vi "csmdoc_list_all_csm_documented_VIs.vi"() -> (3 "Array":path[](array[path]))   [LabVIEW 2017, in "csmdoc.lvlib"]
uses:
  csmdoc.lvlib
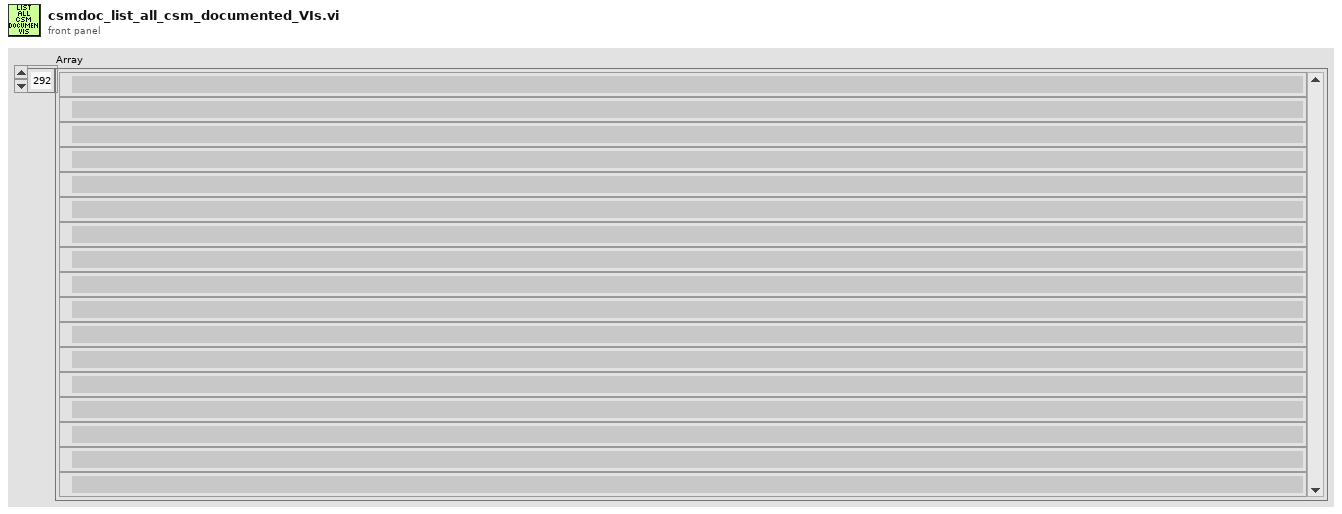
[diagram p1: front panel]
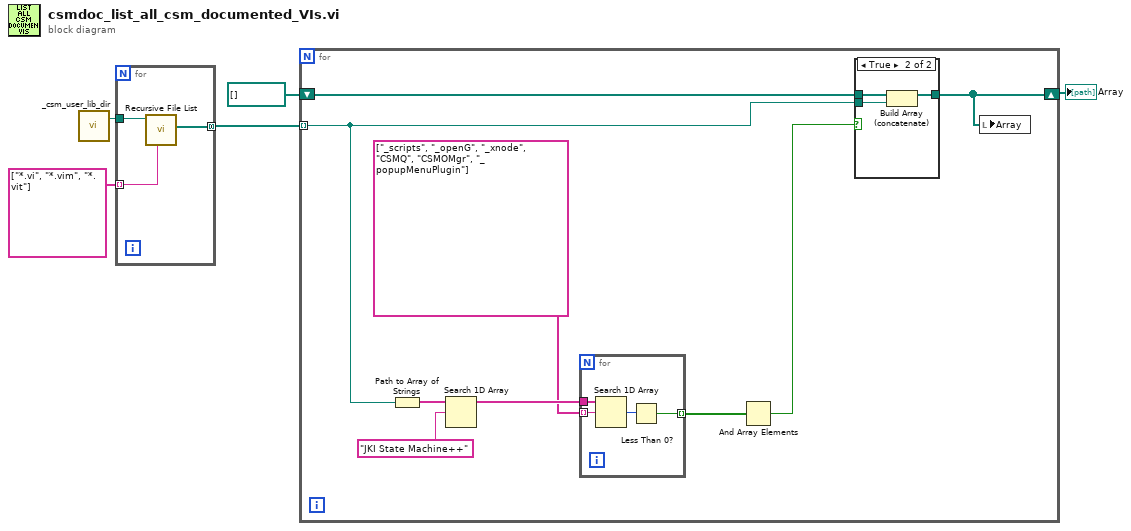
[diagram p0: block diagram]
diagram:
  n1 = call "_csm_user_lib_dir.vi"() -> ("csm_user.lib_dir"=w3:path)  [unwired: 2 in, 1 out]
  n2 = for {
    tunnel: w3 -> [w8]
    tunnel: string[] ["*.vi", "*.vim", "*.vit"] -> [w7] mode=indexing
    tunnel: [w6] -> w4 mode=concatenating
    n3 = call <vilib>:"Recursive File List.vi"("pattern"=w7, "Folder Path"=w8) -> ("All Files in Dir"=w6:path[])  [unwired: 5 in, 4 out]
  }
  n4 = for {
    tunnel: w4 -> [w14] mode=indexing
    shift-right: [w13] -> w1
    shift-left: path[] [] ("All Files in Dir") -> [w15]
    n5 = Path to Array of Strings(0:w14) -> (2:w12:string[])  [unwired: 1 out]
    n6 = Search 1D Array(1D array=w12, element="JKI State Machine++") -> ()  [unwired: 1 in, 1 out]
    n7 = for {
      tunnel: w12 -> [w20]
      tunnel: string[] ["_scripts", "_openG", "_xnode", "CSMQ", "CSMOMgr", "_popupMenuPlugin"] ("element") -> [w19] mode=indexing
      tunnel: [w17] -> w10 mode=indexing
      n8 = Search 1D Array(1D array=w20, element=w19) -> (index of element=w18:i32)  [unwired: 1 in]
      n9 = Less Than 0?(x=w18) -> (x < 0?=w17:bool)
    }
    n10 = And Array Elements(Boolean array=w10) -> (logical AND=w9:bool)
    n11 = case shown="True" w9 {
      tunnel: w15 -> [w21 w24]
      tunnel: [w21 w23] -> w13
      tunnel: w14 -> [_ w22]
      frame False {
      }
      frame True {
        n12 = Build Array (concatenate)(w24, w22) -> (w23:path[])
      }
    }
    n13 = local write "Array"(w13) -> ()
  }
  "Array" <- w1
